vi "Write Setpoint.vi"(8 "error in (no error)":errorcluster, 11 "Bioreactor in":refnum<class "Bioreactor.lvclass">) -> (0 "error out":errorcluster, 3 "Bioreactor out":refnum<class "Bioreactor.lvclass">)   [LabVIEW 2013, in "Bioreactor.lvlib" / "Bioreactor.lvclass"]
uses:
  Bioreactor.lvclass
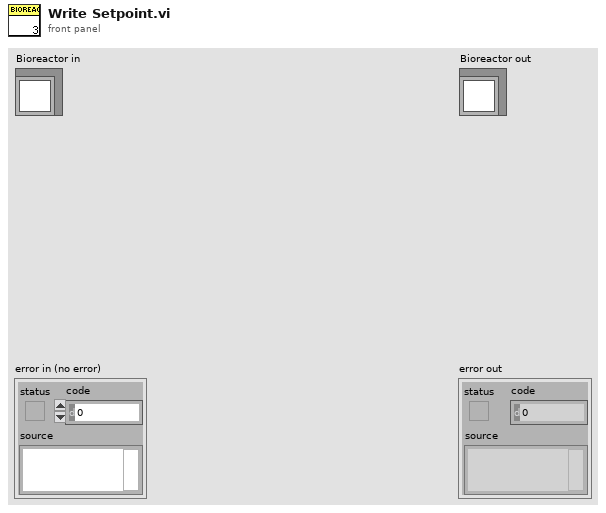
[diagram p1: front panel]
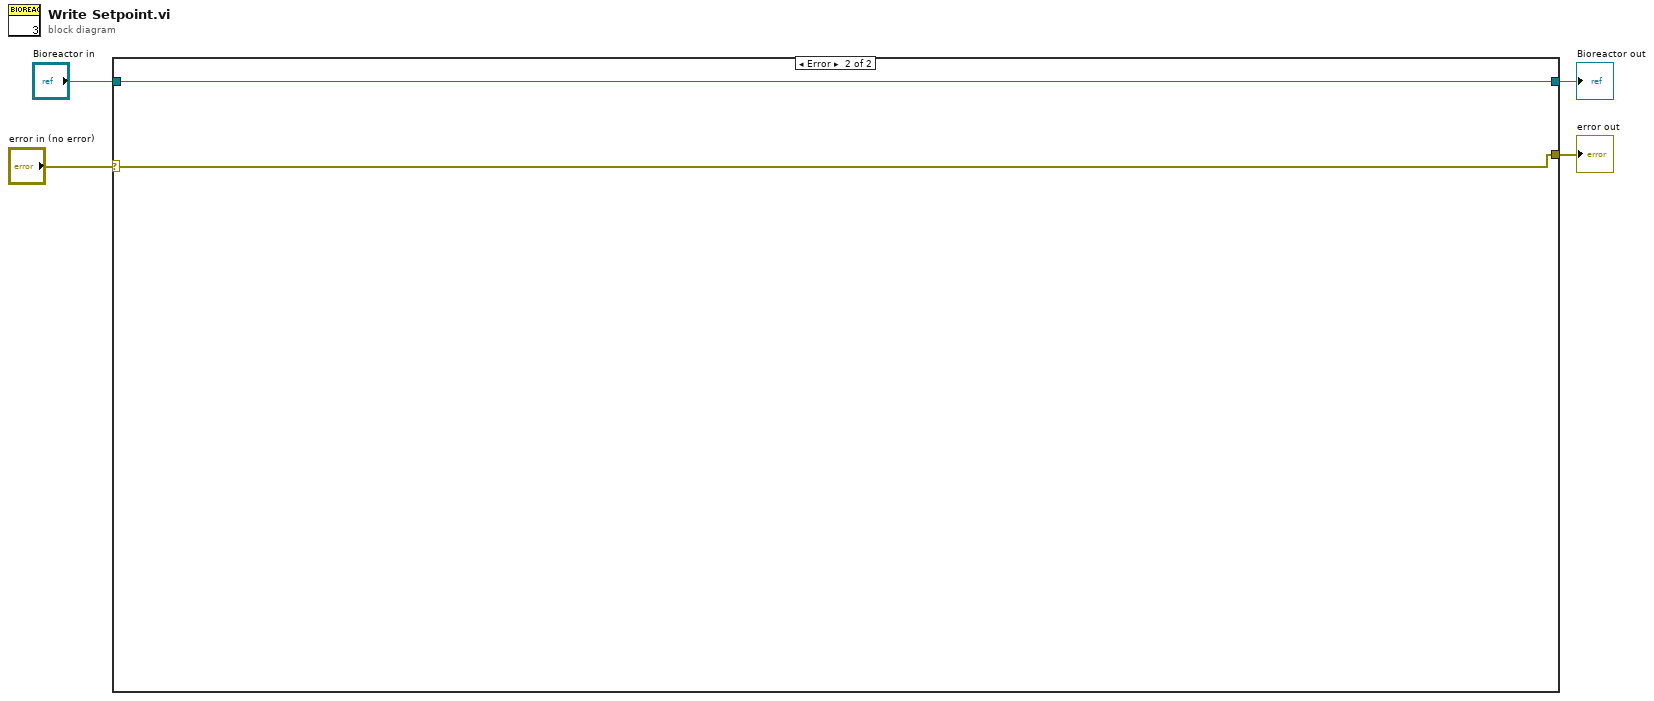
[diagram p0: block diagram]
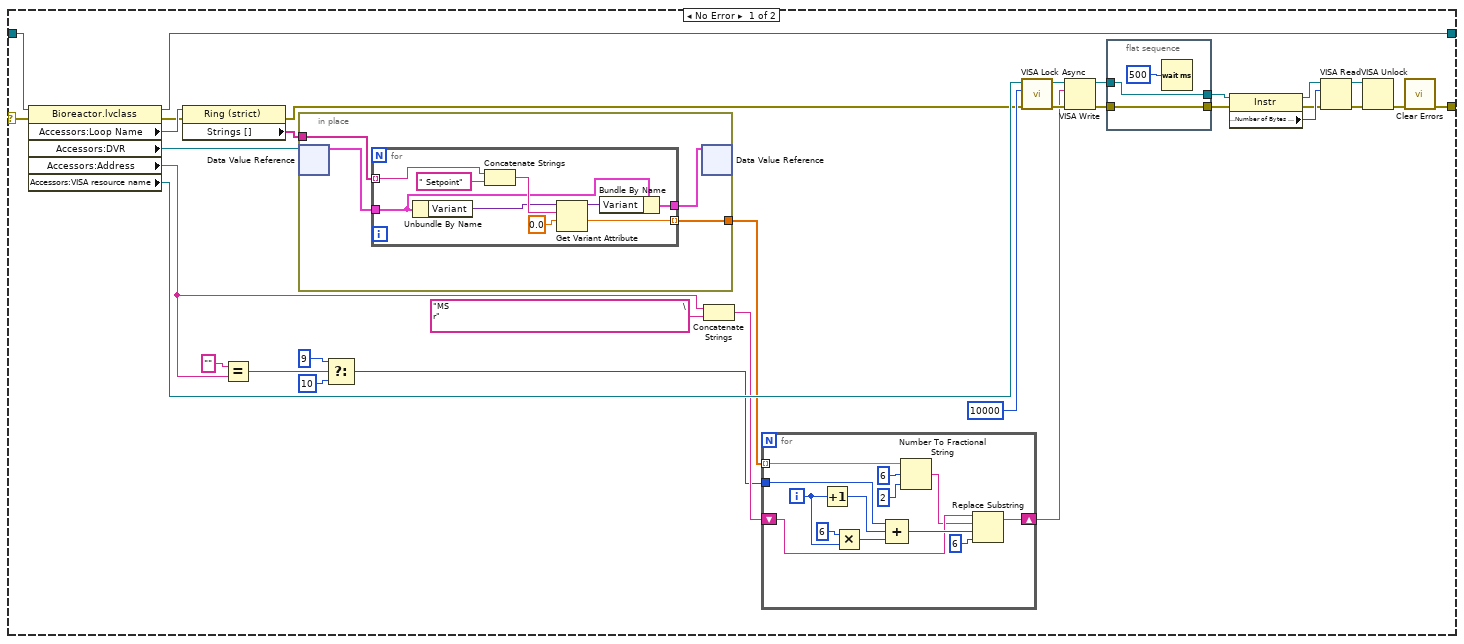
[diagram p2: hidden frame]
diagram:
  n1 = case shown="Error" "error in (no error)" {
    selector: "error in (no error)" -> [w30 w67]
    tunnel: [w7 w68] -> w2
    tunnel: "Bioreactor in" -> [w29 w68]
    tunnel: [w5 w67] -> w1
    frame No Error {
      n2 = property class="Bioreactor.lvclass"(reference=w29, error in=w30) -> (reference out=w7:refnum<class "Bioreactor.lvclass">, error out=w12:errorcluster, "Accessors:Loop Name"=w13:refnum<vi>, "Accessors:DVR"=w10:refnum<data-value>, "Accessors:Address"=w14:string, "Accessors:VISA resource name"=w23:refnum<visa-resource-name>)
      n3 = property class="Ring (strict)"(reference=w13, error in=w12) -> (error out=w11:errorcluster, "Strings []"=w9:string[])  [unwired: 1 out]
      n4 = Equal?(x="", y=w14) -> (x = y?=w19:bool)
      n5 = in-place {
        in-place-border: w9 -> [w41]
        in-place-border: [w38] -> w8
        n6 = in-place-dvr #1(w10) -> (w40:cluster{"Array":string[], "Variant":variant})  [unwired: 1 out]
        n7 = for {
          tunnel: w41 -> [w50] mode=indexing
          tunnel: w40 -> [w45]
          tunnel: [w46] -> w38 mode=indexing
          tunnel: [w42] -> w39
          n8 = Unbundle By Name(w45) -> ("Variant"=w44:variant)
          n9 = Concatenate Strings(w50, " Setpoint" ("string")) -> (w48:string)
          n10 = Get Variant Attribute(Variant=w44, name=w48, default value (empty Variant)=0.0 ("Value")) -> (duplicate Variant=w43:variant, value=w46:dbl)  [unwired: 1 in, 2 out]
          n11 = Bundle By Name(cluster=w45, "Variant"=w43) -> (w42:cluster{"Array":string[], "Variant":variant})
        }
        n12 = in-place-dvr #1(w39) -> ()  [unwired: 2 out]
      }
      n13 = Select(t=9, s=w19, f=10) -> (s? t:f=w15:i32)
      n14 = Concatenate Strings(w14, "MS                                                                              \r" ("y")) -> (w21:string)
      n15 = for {
        tunnel: w15 -> [w63]
        shift-right: [w55] -> w20
        shift-left: w21 -> [w56]
        tunnel: w8 -> [w51] mode=indexing
        i -> [w59]
        n16 = Increment(x=w59) -> (x+1=w61:i32)
        n17 = Multiply(x=6, y=w59) -> (x*y=w58:i32)
        n18 = Compound Arithmetic op=ADD(w63, w61, w58) -> (w62:i32)
        n19 = Number To Fractional String(number=w51, width (-)=i16 6, precision (6)=i16 2 ("width (-)")) -> (F-format string=w52:string)  [unwired: 1 in]
        n20 = Replace Substring(2:6, 3:w62, 4:w52, 5:w56) -> (1:w55:string)  [unwired: 1 out]
      }
      n21 = call <vilib>:"VISA Lock Async.vi"("error in (no error)"=w11, "timeout (0)"=u32 10000, "VISA resource name"=w23) -> ("error out"=w28:errorcluster, "VISA resource name out"=w27:refnum<visa-resource-name>)  [unwired: 6 in, 1 out]
      n22 = VISA Write(VISA resource name=w27, write buffer=w20, error in (no error)=w28) -> (VISA resource name out=w34:refnum<visa-resource-name>, error out=w32:errorcluster)  [unwired: 1 out]
      n23 = flat-sequence {
        tunnel: [w66] -> w33
        tunnel: w34 -> [w66]
        tunnel: [w65] -> w31
        tunnel: w32 -> [w65]
        frame #0 {
          n24 = Wait (ms)(milliseconds to wait=500 ("y")) -> ()  [unwired: 1 out]
        }
      }
      n25 = property class="Instr"(reference=w33, error in=w31) -> (reference out=w35:refnum<visa-resource-name>, error out=w36:errorcluster, "Serial Settings:Number of Bytes at Serial Port"=w37:u32)
      n26 = VISA Read(VISA resource name=w35, byte count=w37, error in (no error)=w36) -> (VISA resource name out=w24:refnum<visa-resource-name>, error out=w25:errorcluster)  [unwired: 2 out]
      n27 = VISA Unlock(8:w25, 11:w24) -> (0:w6:errorcluster)  [unwired: 1 out]
      n28 = call <vilib>:"Clear Errors.vi"("error in (no error)"=w6) -> ("error out"=w5:errorcluster)  [unwired: 6 in]
    }
    frame Error {
    }
  }
  "error out" <- w1
  "Bioreactor out" <- w2
